vi "accept.vi"(8 "error in (no error)":errorcluster, 10 "Visitor":refnum<class "Visitor.lvclass">, 11 "Circle in":refnum<class "Circle.lvclass">) -> (0 "error out":errorcluster, 2 "String":string, 3 "Circle out":refnum<class "Circle.lvclass">)   [LabVIEW 2018, in "Circle.lvclass"]
uses:
  Circle.lvclass
  Visitor Class/Visitor.lvclass
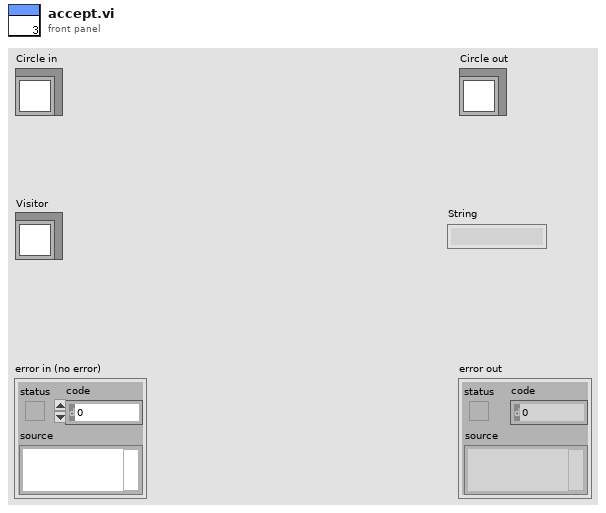
[diagram p1: front panel]
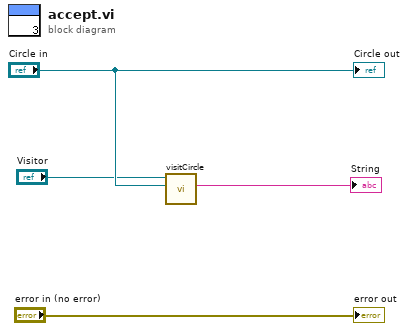
[diagram p0: block diagram]
diagram:
  n1 = call-dynamic "visitCircle.vi"("Circle"="Circle in", "Visitor in"="Visitor") -> ("String"=→"String":string)  [unwired: 7 in, 2 out]
  "error out" <- "error in (no error)"
  "Circle out" <- "Circle in"
